vi "Launch Instruments.vi"(8 "error in":errorcluster, 11 "Controller in":refnum<class "Controller.lvclass">) -> (0 "error out":errorcluster, 3 "Controller out":refnum<class "Controller.lvclass">)   [LabVIEW 2014, in "Controller.lvlib" / "Controller.lvclass"]
doc: "Configure the Instrument objects for operation and stuff them in their appropriate Instr Actor objects, calling their Pre Launch Init methods. The queues for these will be stored in the FGV for communication with the UI."
uses:
  Controller.lvclass
  PAS/Instrument/ePAS.lvclass
  CRDS/Main/eCRDS.lvclass
  FPGA/Session/Exscalabar FPGA.lvclass
  reusable/PAS/Data/Main/PAS Data.lvclass
  Instr Actor/Instr Actor.lvclass
  PAS/Data/Cell/ePAS Cell Data.lvclass
  Update Controller Data MSG.lvclass
  reusable/Instrument/Instrument.lvclass/Instrument.ctl
  PAS/Instrument/ePAS.lvclass/ePAS.ctl
  reusable/DAQ Device/Device/Generic Data Update Data MSG/Generic Update Data Message.lvclass/Generic Update Data Message.ctl
  Instr Actor/Instr Actor.lvclass/Instr Actor.ctl
  SuperActor/Ex Nested.lvclass/Ex Nested.ctl
  reusable/DAQ Device/Device/Generic Data Update Data MSG/Write ID.vi
  Instr Actor/Accessors/Write Instr.vi
  SuperActor/Write ID.vi
  Instr Actor/Accessors/Write Update Data MSG.vi
  reusable/Instrument/Write Data.vi
  PAS/Instrument/Accessors/Write FPGA Session.vi
  reusable/PAS/Data/Main/Write CellData.vi
  <userlib>/_Session Fwk/Session - Root.lvclass
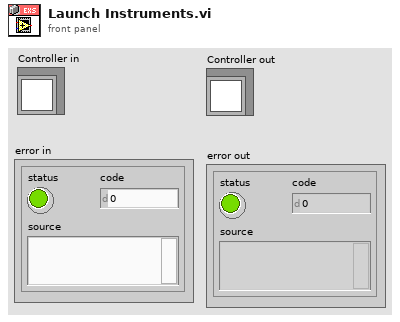
[diagram p1: front panel]
types:
  T1 = typedef "Session - Root.lvclass/Session Handle.ctl" = refnum<data-value>
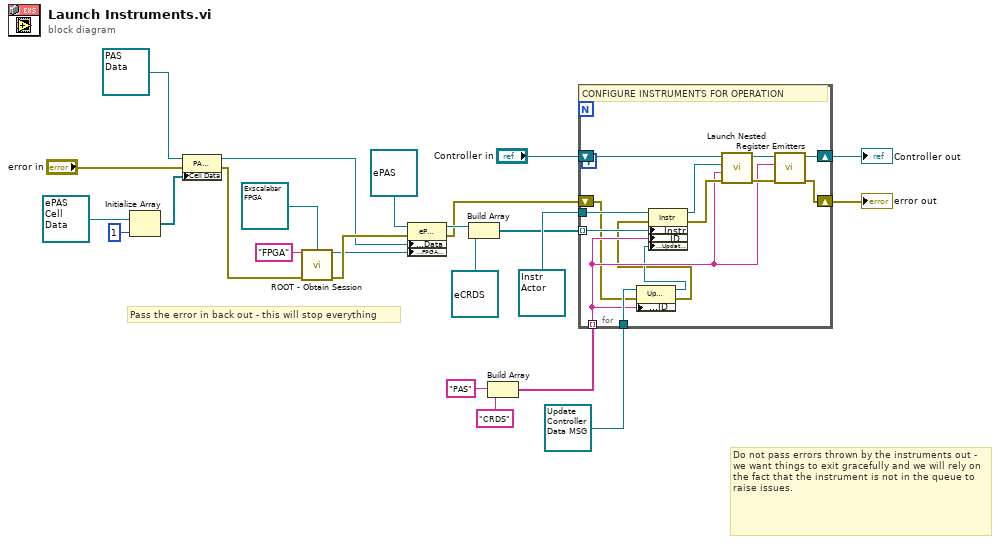
[diagram p0: block diagram]
diagram:
  # "Do not pass errors thrown by the instruments out - we want things to exit gracefully and we will rely on the fact that the instrument is not in the queue to raise issues."
  # "Pass the error in back out - this will stop everything"
  n1 = Initialize Array(refnum<class "ePAS Cell Data.lvclass"> refnum ("ePAS Cell"), 1 ("dimension size")) -> (w21:refnum<class "ePAS Cell Data.lvclass">[])
  n2 = property class="PAS Data"(reference=refnum<class "PAS Data.lvclass"> refnum ("PAS Data"), error in="error in", "Cell Data"=w21) -> (reference out=w11:refnum<class "PAS Data.lvclass">, error out=w22:errorcluster)
  n3 = call <userlib>:"ROOT - Obtain Session.vi"("Session Name ()"="FPGA", "OBJ - Session"=refnum<class "Exscalabar FPGA.lvclass"> refnum ("Ex FPGA"), "error in (no error)"=w22) -> ("Session Handle"=w12:T1, "error out"=w19:errorcluster)  [unwired: 10 in, 1 out]
  n4 = property class="ePAS"(reference=refnum<class "ePAS.lvclass"> refnum ("ePAS.lvclass"), error in=w19, "Accessors:Data"=w11, "Accessors:FPGA Session"=w12) -> (reference out=w18:refnum<class "ePAS.lvclass">, error out=w9:errorcluster)
  n5 = Build Array(w18, refnum<class "eCRDS.lvclass"> refnum ("eCRDS")) -> (w13:refnum<class "Instrument.lvclass">[])
  n6 = Build Array("PAS", "CRDS" ("element")) -> (w6:string[])
  n7 = for {
    tunnel: w13 -> [w38] mode=indexing
    tunnel: refnum<class "Instr Actor.lvclass"> refnum ("Instrument Lib:Instr") -> [w37]
    tunnel: w6 -> [w28] mode=indexing
    shift-right: [w31] -> w4
    shift-left: "Controller in" -> [w36]
    shift-right: [w30] -> w2
    shift-left: w9 -> [w26]
    tunnel: refnum<class "Update Controller Data MSG.lvclass"> refnum ("Controller.lvlib:Update Data MSG") -> [w29]
    # "CONFIGURE INSTRUMENTS FOR OPERATION"
    n8 = property class="Update Data MSG"(reference=w29, error in=w26, "Accessors:ID"=w28) -> (reference out=w27:refnum<class "Update Controller Data MSG.lvclass">, error out=w25:errorcluster)
    n9 = property class="Instr"(reference=w37, error in=w25, "Accessors:Instr"=w38, "Accessors:ID"=w28, "Accessors:Update Data MSG"=w27) -> (reference out=w35:refnum<class "Instr Actor.lvclass">, error out=w34:errorcluster)
    n10 = call "Launch Nested.vi"("Error In"=w34, "ID"=w28, "Nested Actor"=w35, "Controller in"=w36) -> ("Error Out"=w32:errorcluster, "Controller out"=w33:refnum<class "Controller.lvclass">)  [unwired: 6 in]
    n11 = call "Register Emitters.vi"("error in"=w32, "Emitter"=w28, "Controller in"=w33) -> ("error out"=w30:errorcluster, "Controller out"=w31:refnum<class "Controller.lvclass">)  [unwired: 7 in]
  }
  "Controller out" <- w4
  "error out" <- w2
